vi "Create Channel Task.vi"(8 "error in":errorcluster, 10 "SQL query":string="SELECT max(MaximumVoltage),max(MinimumVoltage),max(SampleRate) FROM\nltt.daq_configuration \nWhere ChannelType='PWM_Input' and Enabled=1;", 11 "NI PWM Input in":refnum<class "NI PWM Input.lvclass">) -> (0 "error out":errorcluster, 3 "NI PWM Input out":refnum<class "NI PWM Input.lvclass">)   [LabVIEW 2023, in "HardwareAbstractionLayer_LVOOP.lvlib" / "NI PWM Input.lvclass"]
doc: "This VI Analog Input Voltage Created the Task Physical Channel"
uses:
  NI PWM Input.lvclass
  NI PWM Input.lvclass/NI PWM Input.ctl
  <vilib>/DAQmx/create/channels.llb/DAQmx Create Channel (CI-Pulse Freq).vi
  <vilib>/DAQmx/configure/timing.llb/DAQmx Timing (Implicit).vi
  <resource>/objmgr/daqmx.rc
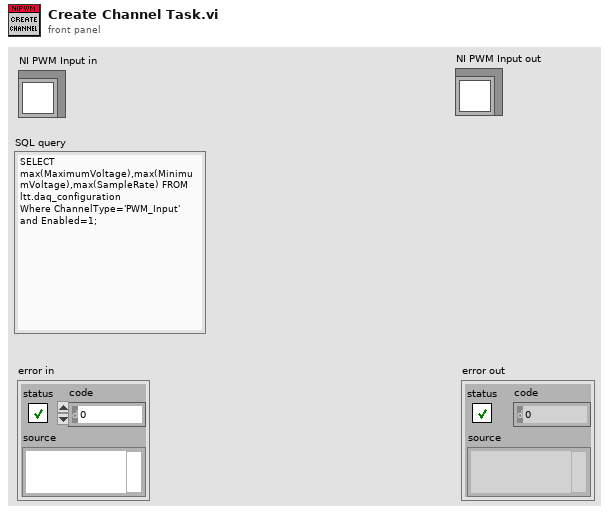
[diagram p1: front panel]
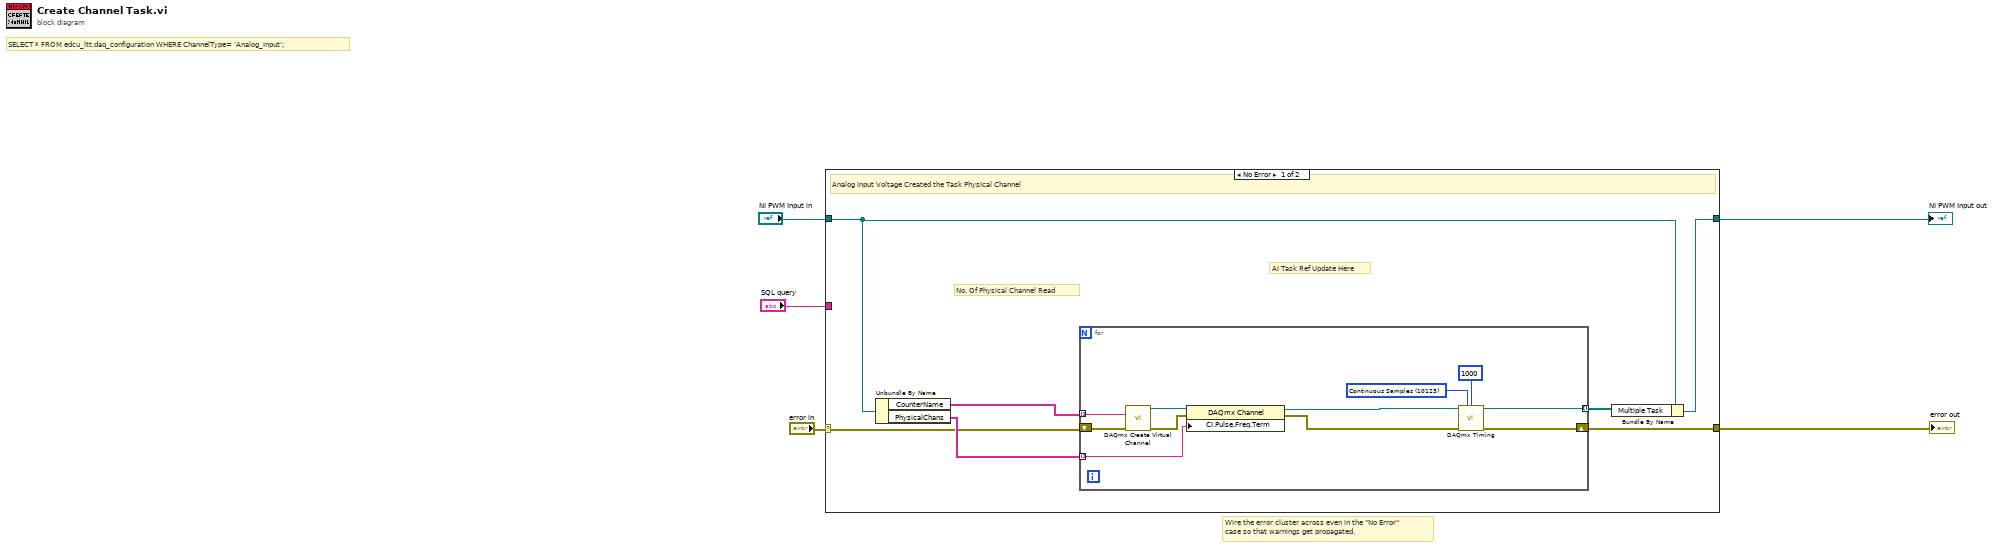
[diagram p0: block diagram]
diagram:
  # "Wire the error cluster across even in the \"No Error\"\ncase so that warnings get propagated."
  # "SELECT * FROM edcu_ltt.daq_configuration WHERE ChannelType= 'Analog_Input';"
  n1 = case shown="No Error" "error in" {
    selector: "error in" -> [w7 w25]
    tunnel: [w10 w25] -> w4
    tunnel: [w11 w24] -> w2
    tunnel: "NI PWM Input in" -> [w12 w24]
    tunnel: "SQL query" -> [_ _]
    frame No Error {
      # "AI Task Ref Update Here"
      # "No. Of Physical Channel Read"
      # "Analog Input Voltage Created the Task Physical Channel"
      n2 = Unbundle By Name(w12) -> ("CounterName"=w8:tag[], "PhysicalChans"=w9:tag[])
      n3 = for {
        tunnel: w9 -> [w15] mode=indexing
        tunnel: w8 -> [w22] mode=indexing
        shift-right: [w16] -> w10
        shift-left: w7 -> [w21]
        tunnel: [w17] -> w6 mode=indexing
        w14 = 10123 items=["Finite Samples"=10178, "Continuous Samples"=10123, "Hardware Timed Single Point"=12522] ("sample mode")
        n4 = call-poly <vilib>:"DAQmx Create Virtual Channel.vi"("counter"=w22, "error in"=w21) -> ("task out"=w20:refnum<k21>, "error out"=w19:errorcluster)  [unwired: 12 in]
        n5 = property class="DAQmx Channel"(reference=w20, error in=w19, "CI.Pulse.Freq.Term"=w15) -> (reference out=w18:refnum<k21>, error out=w23:errorcluster)
        n6 = call-poly <vilib>:"DAQmx Timing.vi"("task/channels in"=w18, "sample mode"=w14, "samples per channel"=1000, "error in"=w23) -> ("task out"=w17:refnum<k21>, "error out"=w16:errorcluster)  [unwired: 10 in]
      }
      n7 = Bundle By Name(cluster=w12, "Multiple Task"=w6) -> (w11:refnum<class "NI PWM Input.lvclass">)
    }
    frame Error {
    }
  }
  "error out" <- w4
  "NI PWM Input out" <- w2
